vi "SignalAdquisition.vi"() -> ()   [LabVIEW 2015]
panel:
  out "x*y 3":dbl[](array[numeric])
  out "x*y 2":dbl[](array[numeric])
  out "x*y":dbl[](array[numeric])
  out "Waveform Graph 3":dbl[](graph)
  out "Waveform Graph 2":dbl[](graph)
  out "transposed array":dbl[][](array[numeric])
  in  "stop (T)":bool=TRUE
  out "Waveform Graph":dbl[](graph)
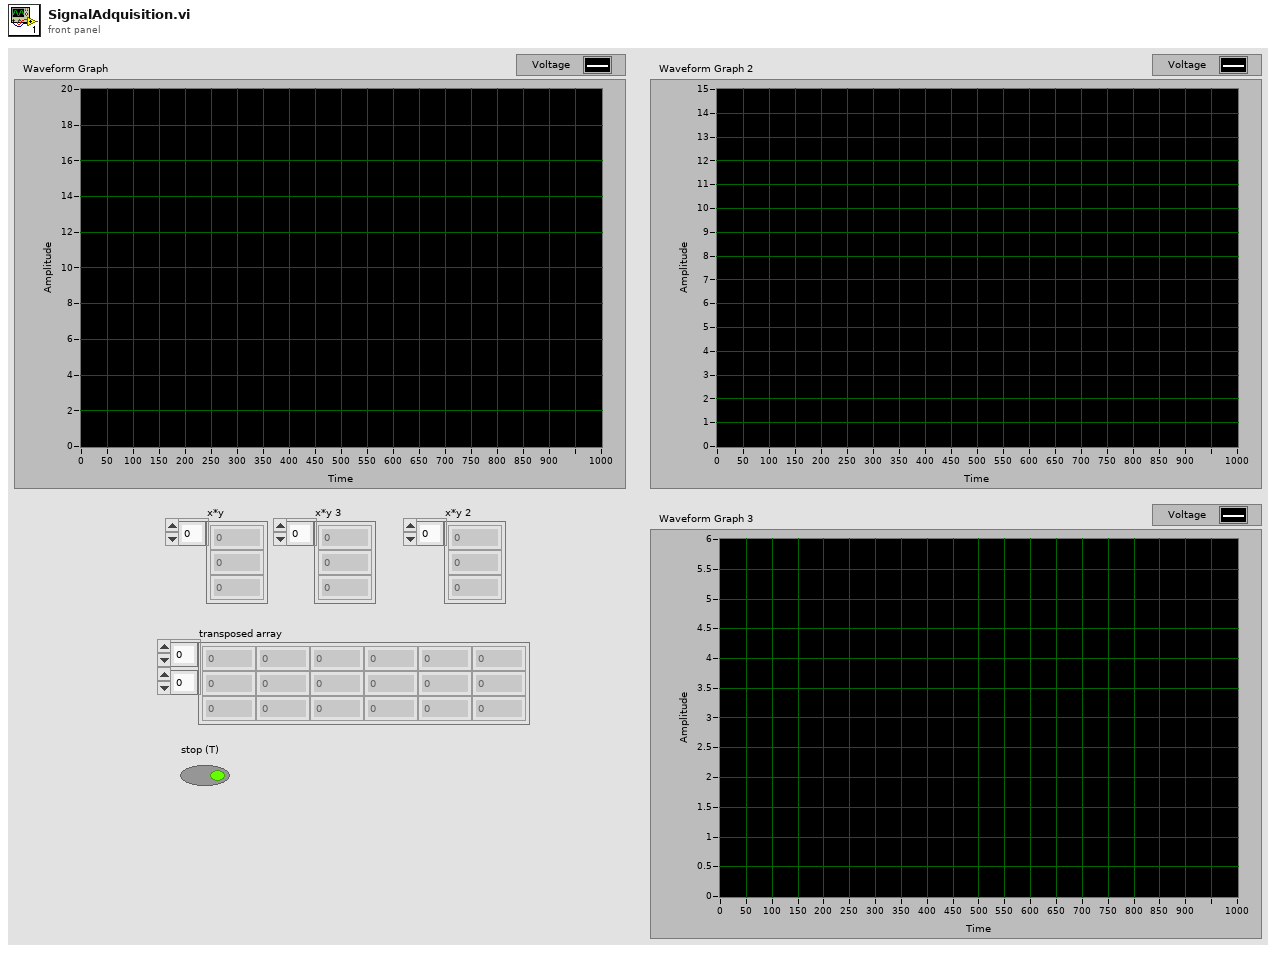
[diagram p1: front panel]
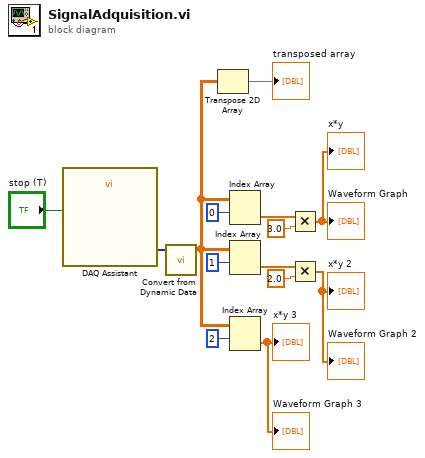
[diagram p0: block diagram]
diagram:
  n1 = call "DAQ Assistant"("stop (T)"="stop (T)") -> ("data"=w13:dynamicdata)  [unwired: 16 in, 2 out]
  n2 = call "Convert from Dynamic Data"("Dynamic Data Type"=w13) -> ("Array"=w8:dbl[][])  [unwired: 3 in]
  n3 = Transpose 2D Array(2D array=w8) -> (transposed array=→"transposed array":dbl[][])
  n4 = Index Array(array=w8, index (row)=0) -> (element=w5:dbl[])  [unwired: 1 in]
  n5 = Index Array(array=w8, index (row)=1) -> (element=w4:dbl[])  [unwired: 1 in]
  n6 = Index Array(array=w8, index (row)=2) -> (element=→"Waveform Graph 3" →"x*y 3":dbl[])  [unwired: 1 in]
  n7 = Multiply(x=w5, y=3.0) -> (x*y=→"Waveform Graph" →"x*y":dbl[])
  n8 = Multiply(x=w4, y=2.0) -> (x*y=→"Waveform Graph 2" →"x*y 2":dbl[])
